vi "CAL-Get Max SPL.vi"(0 "Speaker name":path, 7 "Frequency (kHz)":dbl[](array[numeric]), 11 "error in (no error)":errorcluster) -> (8 "Max SPL":dbl[](array[numeric]), 15 "error out":errorcluster)   [LabVIEW 2020]
uses:
  6e8da5b1-1b00-4d9f-aaf5-506f89b22cd4.vi
  e13087c8-9fd7-40b9-9a87-493df369c5bd.vi
  be18e4bf-d87e-4a2f-b8e4-136f7fe3cc07.vi
panel:
  in  "VDAC":dbl=10.0
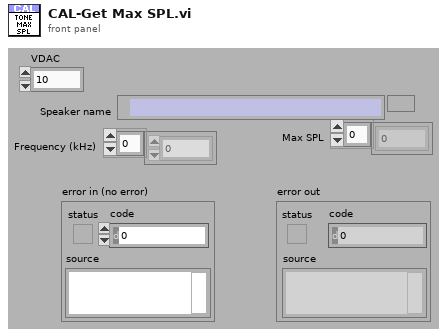
[diagram p1: front panel]
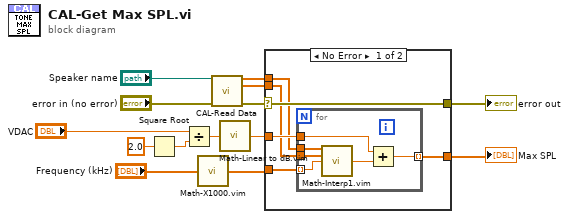
[diagram p0: block diagram]
diagram:
  n1 = Square Root(x=2.0 ("y")) -> (sqrt(x)=w6:dbl)
  n2 = Divide(x="VDAC", y=w6) -> (x/y=w8:dbl)
  n3 = call "Math-X1000.vim"("X"="Frequency (kHz)") -> ("1000X"=w1:dbl[])
  n4 = call "CAL-Read Data.vi"("user path"="Speaker name", "error in (no error)"="error in (no error)") -> ("Frequency (Hz)"=w11:dbl[], "Mag"=w3:dbl[], "error out"=w13:errorcluster)  [unwired: 9 in, 2 out]
  n5 = call "Math-Linear to dB.vim"("linear"=w8) -> ("dB"=w9:dbl)
  n6 = case shown="No Error" w13 {
    selector: w13 -> [w20 w27]
    tunnel: [w20 w27] -> w12
    tunnel: w11 -> [w16 _]
    tunnel: w1 -> [w19 _]
    tunnel: [w18 _] -> w10
    tunnel: w9 -> [w17 _]
    tunnel: w3 -> [w15 _]
    frame No Error {
      n7 = for {
        tunnel: w19 -> [w26] mode=indexing
        tunnel: [w24] -> w18 mode=indexing
        tunnel: w17 -> [w23]
        tunnel: w16 -> [w22]
        tunnel: w15 -> [w21]
        n8 = call "Math-Interp1.vim"("X"=w22, "Y"=w21, "U"=w26) -> ("V"=w25:dbl)  [unwired: 12 in]
        n9 = Add(x=w23, y=w25) -> (x+y=w24:dbl)
      }
    }
    frame Error {
    }
  }
  "error out" <- w12
  "Max SPL" <- w10
